vi "Exercise1BTS.vi"() -> ()   [LabVIEW 2014]
panel:
  out "Result":dbl
  in  "Multiply XY -(T)":bool
  in  "Y":dbl
  in  "X":dbl
  # "Divide X/Y - (T)"
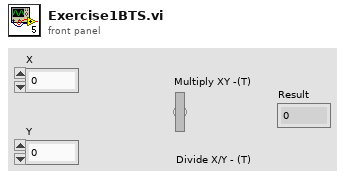
[diagram p1: front panel]
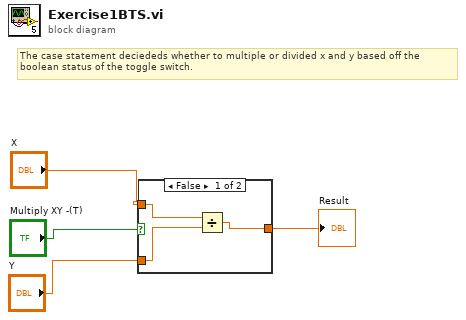
[diagram p0: block diagram]
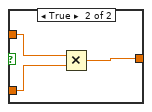
[diagram p2: hidden frame]
diagram:
  # "The case statement deciededs whether to multiple or divided x and y based off the \nboolean status of the toggle switch."
  n1 = case shown="False" "Multiply XY -(T)" {
    tunnel: "Y" -> [w6 w9]
    tunnel: "X" -> [w7 w10]
    tunnel: [w5 w8] -> w1
    frame False {
      n2 = Divide(x=w7, y=w6) -> (x/y=w5:dbl)
    }
    frame True {
      n3 = Multiply(x=w10, y=w9) -> (x*y=w8:dbl)
    }
  }
  "Result" <- w1
